vi "getSheetByName.vi"(8 "error in (no error)":errorcluster, 10 "Sheet Name":string, 11 "MS-Excel in":refnum<class "MS-Excel.lvclass">) -> (0 "error out":errorcluster, 1 "Sheet Ref":refnum<k24>, 2 "SheetIndex":i32, 3 "MS-Excel out":refnum<class "MS-Excel.lvclass">)   [LabVIEW 2020, in "LabVIEW NPOI.lvlib" / "MS-Excel.lvclass"]
doc: "Returns the <b>SheetIndex</b> and the <b>SheetI Ref</b> of the sheet nammed <b>Sheet Name</b>."
uses:
  MS-Excel.lvclass
  D:/Benjamin/Documents/Perso/Code/WC/LabVIEW_NPOI/lib/NPOI 2.1.1/NPOI.dll
  lib/NPOI 2.1.1/NPOI.dll
  MS-Excel.lvclass/MS-Excel.ctl
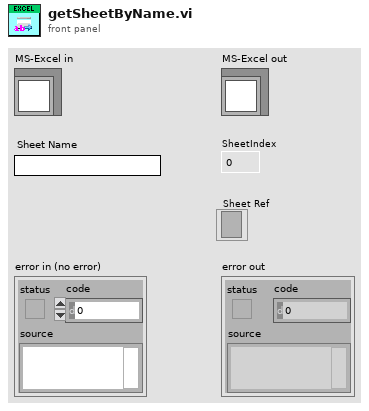
[diagram p1: front panel]
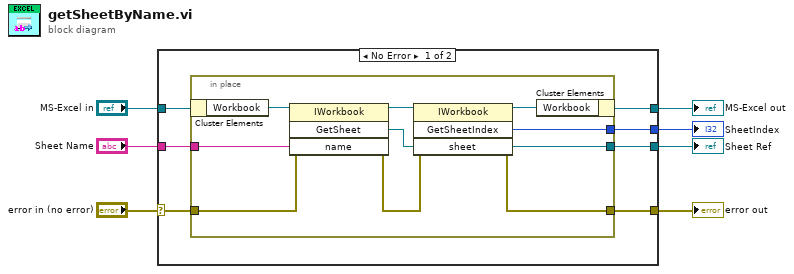
[diagram p0: block diagram]
diagram:
  n1 = case shown="No Error" "error in (no error)" {
    selector: "error in (no error)" -> [w11 w24]
    tunnel: [w10 w24] -> w7
    tunnel: [w14 w25] -> w5
    tunnel: "MS-Excel in" -> [w13 w25]
    tunnel: "Sheet Name" -> [w12 _]
    tunnel: [w9 _] -> w2
    tunnel: [w8 _] -> w1
    frame No Error {
      n2 = in-place {
        in-place-border: w12 -> [w22]
        in-place-border: w11 -> [w21]
        in-place-border: [w17] -> w10
        in-place-border: [w15] -> w9
        in-place-border: [w16] -> w8
        n3 = in-place-cluster #1(w13) -> ("Workbook"=w23:refnum<k24>)
        n4 = invoke class="IWorkbook" method="GetSheet"(reference=w23, error in=w21, "name"=w22) -> (reference out=w20:refnum<k24>, error out=w18:errorcluster, "GetSheet"=w15:refnum<k24>)  [unwired: 1 in, 1 out]
        n5 = invoke class="IWorkbook" method="GetSheetIndex"(reference=w20, error in=w18, "sheet"=w15) -> (reference out=w19:refnum<k24>, error out=w17:errorcluster, "GetSheetIndex"=w16:i32)  [unwired: 1 in, 1 out]
        n6 = in-place-cluster #1("Workbook"=w19) -> (w14:refnum<class "MS-Excel.lvclass">)
      }
    }
    frame Error {
    }
  }
  "error out" <- w7
  "MS-Excel out" <- w5
  "Sheet Ref" <- w2
  "SheetIndex" <- w1
